vi "WLAN_STF.vi"() -> (3 "STF":cdb[](array[numeric]))   [LabVIEW 2014]
uses:
  <vilib>/Analysis/2dsp.llb/Inverse Complex FFT.vi
  <vilib>/Analysis/NI_AALPro.lvlib
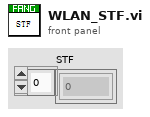
[diagram p1: front panel]
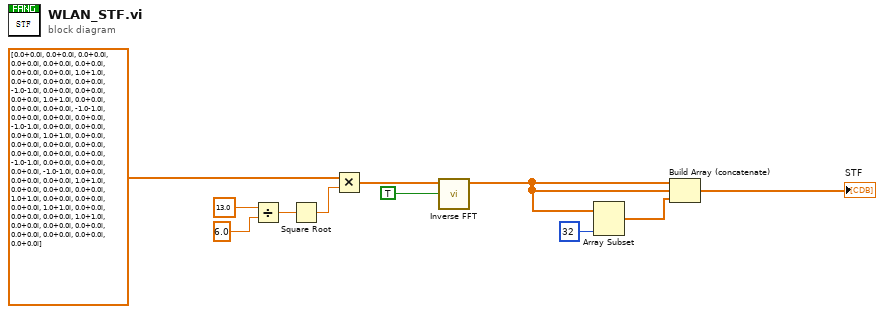
[diagram p0: block diagram]
diagram:
  n1 = Divide(x=13.0, y=6.0) -> (x/y=w8:dbl)
  n2 = Square Root(x=w8) -> (sqrt(x)=w7:dbl)
  n3 = Multiply(x=cdb[] [0.0+0.0i, 0.0+0.0i, 0.0+0.0i, 0.0+0.0i, 0.0+0.0i, 0.0+0.0i, 0.0+0.0i, 0.0+0.0i, 1.0+1.0i, 0.0+0.0i, 0.0+0.0i, 0.0+0.0i, -1.0-1.0i, 0.0+0.0i, 0.0+0.0i, 0.0+0.0i, 1.0+1.0i, 0.0+0.0i, 0.0+0.0i, 0.0+0.0i, -1.0-1.0i, 0.0+0.0i, 0.0+0.0i, 0.0+0.0i, -1.0-1.0i, 0.0+0.0i, 0.0+0.0i, 0.0+0.0i, 1.0+1.0i, 0.0+0.0i, 0.0+0.0i, 0.0+0.0i, 0.0+0.0i, 0.0+0.0i, 0.0+0.0i, 0.0+0.0i, -1.0-1.0i, 0.0+0.0i, 0.0+0.0i, 0.0+0.0i, -1.0-1.0i, 0.0+0.0i, 0.0+0.0i, 0.0+0.0i, 1.0+1.0i, 0.0+0.0i, 0.0+0.0i, 0.0+0.0i, 1.0+1.0i, 0.0+0.0i, 0.0+0.0i, 0.0+0.0i, 1.0+1.0i, 0.0+0.0i, 0.0+0.0i, 0.0+0.0i, 1.0+1.0i, 0.0+0.0i, 0.0+0.0i, 0.0+0.0i, 0.0+0.0i, 0.0+0.0i, 0.0+0.0i, 0.0+0.0i], y=w7) -> (x*y=w5:cdb[])
  n4 = call-poly <vilib>:"Inverse FFT.vi"("shift?"=TRUE, "FFT {X}"=w5) -> ("X"=w1:cdb[])  [unwired: 8 in, 1 out]
  n5 = Array Subset(array=w1, length=32) -> (w3:cdb[])  [unwired: 1 in]
  n6 = Build Array (concatenate)(w1, w1, w3) -> (→"STF":cdb[])
